vi "toml_example_datatypes.vi"() -> ()   [LabVIEW 2017]
uses:
  b840e024-a058-4075-b0d4-c9d64e0cf193.vi
  toml/toml.llb/toml_value_boolean.vi
panel:
  out "error out":errorcluster
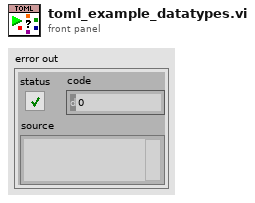
[diagram p1: front panel]
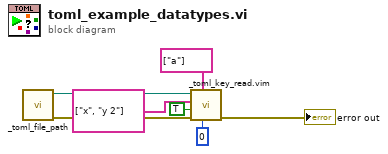
[diagram p0: block diagram]
diagram:
  n1 = call "_toml_file_path.vi"() -> ("error out"=w1:errorcluster, "app toml path"=w6:path)  [unwired: 8 in, 2 out]
  n2 = call "_toml_key_read.vim"("modifiers"=u16 0, "section [str,1d,pth]"=string[] ["a"] ("section"), "error in (no error)"=w1, "default [any]"=TRUE ("default"), "key [str,1d,pth]"=string[] ["x", "y 2"] ("key"), "path in"=w6) -> ("error out"=→"error out":errorcluster)  [unwired: 2 in, 3 out]
